vi "SSC DCPower Configure Settings Array.vi"(0 "DCPower SSC in":T3[](array[typedef]), 1 "Aperture Time Units":T2[](array[typedef]) items=["Seconds"=1028, "Powerline Cycles"=1029], 2 "Transient Response":i32[](array[ring]) items=["Slow"=1041, "Normal"=1038, "Fast"=1039, "Custom"=1042], 5 "Aperture Time":dbl[](array[numeric]) format="%#_6p", 7 "Source Delay (s)":dbl[](array[numeric]) format="%#_6p", 9 "Sense":T1[](array[typedef]) items=["Local"=1008, "Remote"=1009], 11 "error in":errorcluster) -> (4 "DCPower SSC out":T3[](array[typedef]), 15 "error out":errorcluster)   [LabVIEW 2019]
doc: "This VI configures important DCPower channel settings for the sessions.\n\nSettings are ignored if they aren't supported by the device being used.\n\nNote all inputs are required, and all need to be populated with values for every session."
uses:
  SSC DCPower.ctl
  <instrlib>/niDCPower/nidcpower.llb/niDCPower Aperture Time Units.ctl
  <instrlib>/niDCPower/nidcpower.llb/niDCPower Sense.ctl
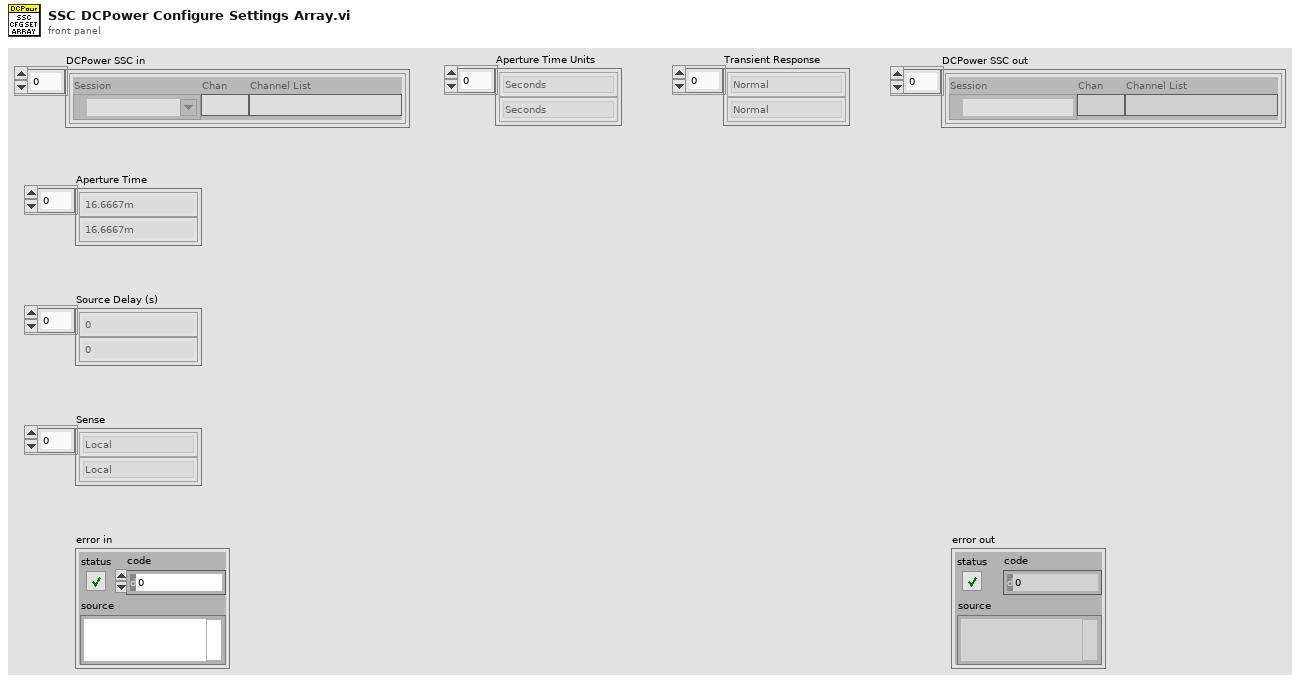
[diagram p1: front panel]
types:
  T1 = typedef "niDCPower Sense.ctl" = i32
  T2 = typedef "niDCPower Aperture Time Units.ctl" = i32
  T3 = typedef "SSC DCPower.ctl" = cluster{"Session":refnum<k15>, "Chan":string, "Channel List":string}
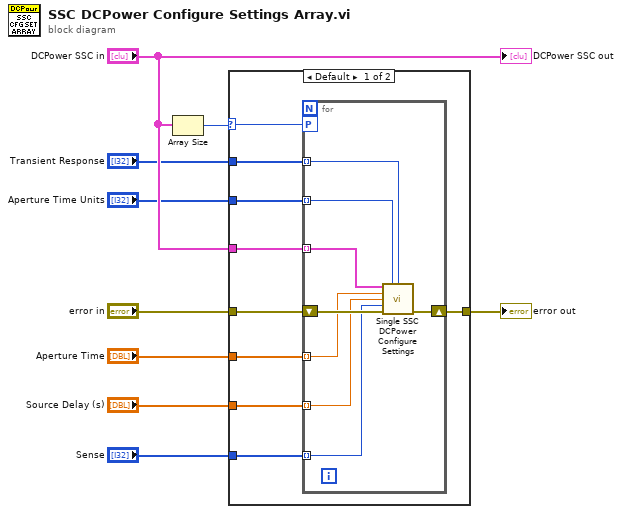
[diagram p0: block diagram]
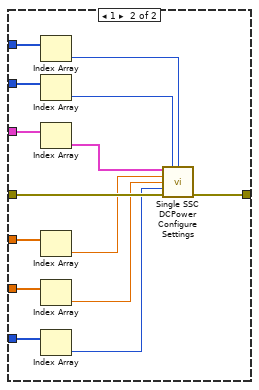
[diagram p2: hidden frame]
diagram:
  n1 = Array Size(array="DCPower SSC in") -> (size(s)=w7:i32)
  n2 = case shown="Default" w7 {
    selector: w7 -> [w16 _]
    tunnel: "error in" -> [w18 w40]
    tunnel: [w17 w39] -> w8
    tunnel: "DCPower SSC in" -> [w15 w38]
    tunnel: "Aperture Time Units" -> [w14 w37]
    tunnel: "Transient Response" -> [w13 w36]
    tunnel: "Aperture Time" -> [w12 w35]
    tunnel: "Source Delay (s)" -> [w11 w34]
    tunnel: "Sense" -> [w10 w33]
    frame Default {
      n3 = for {
        workers-P: w16 -> [_]
        shift-right: [w25] -> w17
        shift-left: w18 -> [w26]
        tunnel: w15 -> [w24] mode=indexing
        tunnel: w14 -> [w23] mode=indexing
        tunnel: w13 -> [w22] mode=indexing
        tunnel: w12 -> [w21] mode=indexing
        tunnel: w11 -> [w20] mode=indexing
        tunnel: w10 -> [w19] mode=indexing
        n4 = call "Single SSC DCPower Configure Settings.vi"("DCPower SSC in"=w24, "Aperture Time Units (Seconds)"=w23, "Transient Response (Normal)"=w22, "Aperture Time (16.6m)"=w21, "Source Delay (0 seconds)"=w20, "Sense (Local)"=w19, "error in"=w26) -> ("error out"=w25:errorcluster)  [unwired: 7 in, 1 out]
      }
    }
    frame 1 {
      n5 = Index Array(array=w36) -> (element=w32:i32)  [unwired: 1 in]
      n6 = Index Array(array=w37) -> (element=w31:T2)  [unwired: 1 in]
      n7 = Index Array(array=w38) -> (element=w30:T3)  [unwired: 1 in]
      n8 = Index Array(array=w35) -> (element=w29:dbl)  [unwired: 1 in]
      n9 = Index Array(array=w34) -> (element=w28:dbl)  [unwired: 1 in]
      n10 = Index Array(array=w33) -> (element=w27:T1)  [unwired: 1 in]
      n11 = call "Single SSC DCPower Configure Settings.vi"("DCPower SSC in"=w30, "Aperture Time Units (Seconds)"=w31, "Transient Response (Normal)"=w32, "Aperture Time (16.6m)"=w29, "Source Delay (0 seconds)"=w28, "Sense (Local)"=w27, "error in"=w40) -> ("error out"=w39:errorcluster)  [unwired: 7 in, 1 out]
    }
  }
  "error out" <- w8
  "DCPower SSC out" <- "DCPower SSC in"
